vi "CompareAnkleRange.vi"(6 "Direction(x)":T2, 8 "Minimal Ankle Range":dbl, 9 "AnkleTrajSoFar":dbl[][](array[numeric]), 10 "AnklePosCurrent":dbl[](array[numeric]), 11 "Gait Phase":T1=enum."Stance") -> (3 "Range Greator than Minimum":bool)   [LabVIEW 2016, in "ForceField.lvclass"]
uses:
  ForceField.lvclass
  SerialChain/TypeDef/xyzO.ctl
  TypeDef/GaitPhase.ctl
  SerialChain/SerialChain.lvclass
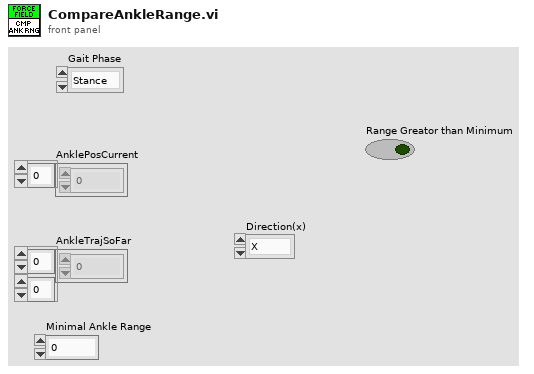
[diagram p1: front panel]
types:
  T1 = typedef "ForceField.lvclass/GaitPhase.ctl" = enum16{"HeelStrk", "Stance", "ToeOff", "Swing"}
  T2 = typedef "SerialChain.lvclass/xyzO.ctl" = enum16{"X", "Y", "Z", "O"}
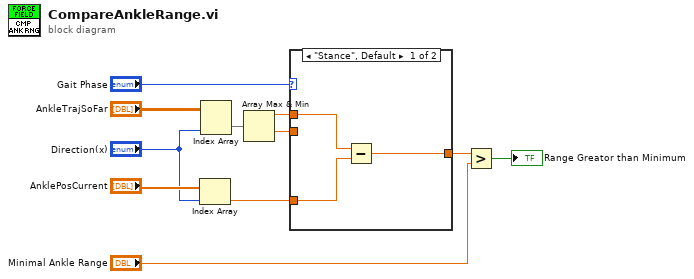
[diagram p0: block diagram]
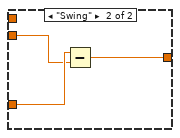
[diagram p2: hidden frame]
diagram:
  n1 = Index Array(array="AnklePosCurrent", index="Direction(x)") -> (element=w3:dbl)
  n2 = Index Array(array="AnkleTrajSoFar", index (col)="Direction(x)") -> (element=w7:dbl[])  [unwired: 1 in]
  n3 = Array Max & Min(array=w7) -> (max value=w6:dbl, min value=w5:dbl)  [unwired: 2 out]
  n4 = case shown="\"Stance\", Default" "Gait Phase" {
    tunnel: w6 -> [w14 _]
    tunnel: w5 -> [_ w15]
    tunnel: w3 -> [w13 w16]
    tunnel: [w12 w17] -> w2
    frame "Stance", Default {
      n5 = Subtract(x=w14, y=w13) -> (x-y=w12:dbl)
    }
    frame "Swing" {
      n6 = Subtract(x=w16, y=w15) -> (x-y=w17:dbl)
    }
  }
  n7 = Greater?(x=w2, y="Minimal Ankle Range") -> (0:→"Range Greator than Minimum":bool)
